vi "To XML (Core).vi"(8 "error in (no error)":errorcluster, 10 "Parent":refnum<k20>, 11 "Test Case in":refnum<class "Test Case.lvclass">) -> (0 "error out":errorcluster)   [LabVIEW 2013, in "JUnit XML.lvlib" / "Test Case.lvclass"]
doc: "Serializes a Test Case using NI XML Parser."
uses:
  Test Case.lvclass
  Test Case.lvclass/Test Case.ctl
  <vilib>/xml/Close Reference(Node).vi
  <vilib>/xml/NI_XML.lvlib
  JUnit XML.lvlib
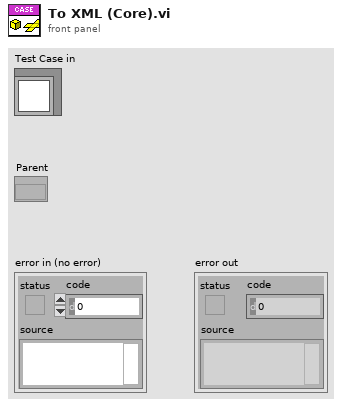
[diagram p1: front panel]
types:
  T1 = typedef "JUnit XML.lvlib/Test Case.lvclass/Test Result.ctl" = enum16{"Success", "Failure", "Error", "Skipped"}
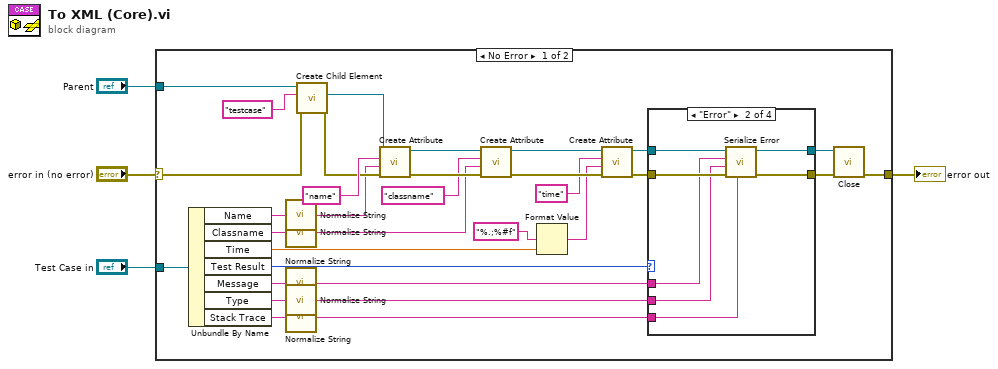
[diagram p0: block diagram]
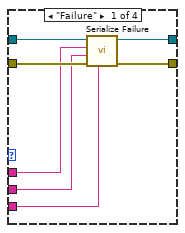
[diagram p2: hidden frame]
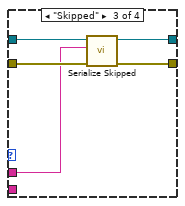
[diagram p3: hidden frame]
diagram:
  n1 = case shown="No Error" "error in (no error)" {
    selector: "error in (no error)" -> [w13 w58]
    tunnel: [w12 w58] -> w3
    tunnel: "Test Case in" -> [w11 _]
    tunnel: "Parent" -> [w10 _]
    frame No Error {
      n2 = Unbundle By Name(w11) -> ("Name"=w34:string, "Classname"=w24:string, "Time"=w23:dbl, "Test Result"=w21:T1, "Message"=w18:string, "Type"=w17:string, "Stack Trace"=w14:string)
      n3 = call "Normalize String.vi"("String"=w34) -> ("Normalized String"=w9:string)  [unwired: 1 in]
      n4 = call "Normalize String.vi"("String"=w24) -> ("Normalized String"=w8:string)  [unwired: 1 in]
      n5 = call "Normalize String.vi"("String"=w18) -> ("Normalized String"=w6:string)  [unwired: 1 in]
      n6 = call "Normalize String.vi"("String"=w17) -> ("Normalized String"=w7:string)  [unwired: 1 in]
      n7 = call "Normalize String.vi"("String"=w14) -> ("Normalized String"=w5:string)  [unwired: 1 in]
      n8 = call "Create Child Element.vi"("error in (no error)"=w13, "Name"="testcase" ("Tag Name"), "Node in"=w10) -> ("error out"=w25:errorcluster, "Child Element"=w26:refnum<k20>)  [unwired: 6 in, 1 out]
      n9 = call "Create Attribute.vi"("error in (no error)"=w25, "Value"=w9, "Name"="name" ("Attribute Name"), "Element in"=w26) -> ("error out"=w32:errorcluster, "Element out"=w33:refnum<k20>)  [unwired: 6 in]
      n10 = call "Create Attribute.vi"("error in (no error)"=w32, "Value"=w8, "Name"="classname" ("Attribute Name"), "Element in"=w33) -> ("error out"=w29:errorcluster, "Element out"=w30:refnum<k20>)  [unwired: 6 in]
      n11 = Format Value(format string="%.;%#f", value (0)=w23) -> (output string=w22:string)  [unwired: 1 in]
      n12 = call "Create Attribute.vi"("error in (no error)"=w29, "Value"=w22, "Name"="time" ("Attribute Name"), "Element in"=w30) -> ("error out"=w15:errorcluster, "Element out"=w16:refnum<k20>)  [unwired: 6 in]
      n13 = case shown="\"Error\"" w21 {
        tunnel: w16 -> [w43 w50 w55 w57]
        tunnel: [w42 w49 w54 w57] -> w20
        tunnel: [w41 w48 w53 w56] -> w19
        tunnel: w15 -> [w40 w47 w52 w56]
        tunnel: w6 -> [w39 w46 w51 _]
        tunnel: w7 -> [w38 w45 _ _]
        tunnel: w5 -> [w37 w44 _ _]
        frame "Failure" {
          n14 = call "Serialize Failure.vi"("Stack Trace"=w37, "error in (no error)"=w40, "Type"=w38, "Message"=w39, "Node in"=w43) -> ("error out"=w41:errorcluster, "Node out"=w42:refnum<k20>)  [unwired: 5 in]
        }
        frame "Error" {
          n15 = call "Serialize Error.vi"("Stack Trace"=w44, "error in (no error)"=w47, "Type"=w45, "Message"=w46, "Node in"=w50) -> ("error out"=w48:errorcluster, "Node out"=w49:refnum<k20>)  [unwired: 5 in]
        }
        frame "Skipped" {
          n16 = call "Serialize Skipped.vi"("error in (no error)"=w52, "Message"=w51, "Node in"=w55) -> ("error out"=w53:errorcluster, "Node out"=w54:refnum<k20>)  [unwired: 7 in]
        }
        frame "Success" {
        }
      }
      n17 = call-poly <vilib>:"Close.vi"("error in (no error)"=w19, "node"=w20) -> ("error out"=w12:errorcluster)  [unwired: 7 in]
    }
    frame Error {
    }
  }
  "error out" <- w3
